vi "RT Train PID.vi"() -> ()   [LabVIEW 2018]
uses:
  <vilib>/Platform/TimedLoop/XDataNode/timing_clust.ctl
  <vilib>/Platform/TimedLoop/XDataNode/nitl_modes.ctl
  <vilib>/Platform/TimedLoop/XDataNode/wakeup.ctl
  <vilib>/Analysis/3filter.llb/Filter Passband Type.ctl
  <vilib>/myRIO/Instrument Drivers/Onboard IO/AI/typedefs/AI Reference.ctl
  <vilib>/myRIO/Common/Instrument Driver Framework/Utilities/typedefs/myRIO Generic Hardware Reference.ctl
  <vilib>/myRIO/Common/Instrument Driver Framework/Utilities/typedefs/Hardware Version Enum.ctl
  <vilib>/myRIO/Common/Instrument Driver Framework/Utilities/typedefs/myRIO v1.0 Reference.ctl
  <vilib>/myRIO/Common/Instrument Driver Framework/Utilities/typedefs/Generic FPGA Reference.ctl
  <vilib>/myRIO/Common/Instrument Driver Framework/myRIO v1.0/AI/typedefs/AI Channels List.ctl
  <vilib>/myRIO/Common/Instrument Driver Framework/myRIO v1.0/AI/typedefs/AI Channels Enum.ctl
  <vilib>/myRIO/Common/Instrument Driver Framework/Utilities/typedefs/Analog Scaling Constants List.ctl
  <vilib>/myRIO/Common/Instrument Driver Framework/Utilities/typedefs/Analog Scaling Constants.ctl
  <vilib>/userdefined/High Color/nirio_resource_hc.ctl
  <vilib>/myRIO/Instrument Drivers/Onboard IO/AO/typedefs/AO Reference.ctl
  <vilib>/myRIO/Common/Instrument Driver Framework/myRIO v1.0/AO/typedefs/AO Channels List.ctl
  <vilib>/myRIO/Common/Instrument Driver Framework/myRIO v1.0/AO/typedefs/AO Channels Enum.ctl
  <vilib>/myRIO/Common/Instrument Driver Framework/Utilities/vis/Is FPGA Ref Available.vi
  <vilib>/myRIO/Common/Instrument Driver Framework/ELVIS III v1.0/AI/vis/ELVIS III v1.1 Open AI.vi
  <vilib>/myRIO/Instrument Drivers/Onboard IO/AI/vis/Read.vi
  6108935b-3925-4b35-9418-db60e5ea9904.vi
  <vilib>/myRIO/Common/Instrument Driver Framework/ELVIS III v1.0/AO/vis/ELVIS III v1.1 Open AO.vi
  <vilib>/myRIO/Instrument Drivers/Onboard IO/AO/vis/Write.vi
  <vilib>/myRIO/Common/Instrument Driver Framework/Utilities/vis/Validate Channels.vi
  <vilib>/myRIO/Common/Instrument Driver Framework/ELVIS III v1.0/AI/vis/ELVIS III v1.0 Reserve AI.vi
  <vilib>/myRIO/Common/Instrument Driver Framework/ELVIS III v1.0/AO/vis/ELVIS III v1.0 Reserve AO.vi
  <vilib>/myRIO/Common/Instrument Driver Framework/ELVIS III v1.0/Resource Manager/vis/ELVIS III v1.0 Reserve Channel List.vi
  <vilib>/myRIO/Common/Instrument Driver Framework/ELVIS III v1.0/AI/vis/ELVIS III v1.0 Build MUX Configuration AI.vi
  <vilib>/myRIO/Common/Instrument Driver Framework/ELVIS III v1.0/AO/vis/ELVIS III v1.0 Build MUX Configuration AO.vi
  <vilib>/myRIO/Common/Instrument Driver Framework/ELVIS III v1.0/Resource Manager/vis/ELVIS III v1.0 Reserve Channel.vi
  <vilib>/myRIO/Common/Instrument Driver Framework/ELVIS III v1.0/Resource Manager/vis/ELVIS III v1.0 Unreserve Channel.vi
  <vilib>/myRIO/Common/Instrument Driver Framework/ELVIS III v1.0/Resource Manager/vis/ELVIS III v1.0 Build Mutex Name.vi
  <vilib>/Utility/VariantDataType/GetNumericInfo.vi
  <vilib>/Utility/error.llb/Error Cluster From Error Code.vi
  <vilib>/myRIO/Common/Instrument Driver Framework/ELVIS III v1.0/ELVIS III v1.1 Open.vi
  <vilib>/myRIO/Common/Instrument Driver Framework/Utilities/vis/IO Manager.vi
  <vilib>/myRIO/Common/Instrument Driver Framework/Utilities/vis/Configuration Manager.vi
  <vilib>/myRIO/Common/Instrument Driver Framework/myRIO v1.0/myRIO v1.0 Close.vi
  <vilib>/myRIO/Common/Instrument Driver Framework/ELVIS III v1.0/AO/vis/ELVIS III v1.0 Write AO.vi
  <vilib>/addons/control/pid/pid.llb/PID (DBL).vi
  <vilib>/myRIO/Common/Instrument Driver Framework/ELVIS III v1.0/Resource Manager/vis/ELVIS III v1.0 Coerce AI Scaling.vi
  <vilib>/myRIO/Common/Instrument Driver Framework/ELVIS III v1.0/Resource Manager/vis/ELVIS III v1.0 Configure AI Mode.vi
  <vilib>/myRIO/Common/Instrument Driver Framework/ELVIS III v1.0/AI/vis/ELVIS III v1.0 Read AI.vi
  <vilib>/myRIO/Express VI/Onboard IO/AO/AO Express VI.xnode
  <vilib>/myRIO/Instrument Drivers/Onboard IO/AO/vis/myRIO AO Open.xnode
  <vilib>/platform/TimedLoop/XDataNode/XDataNode.xnode
  <vilib>/myRIO/Express VI/Onboard IO/AI/AI Express VI.xnode
  <vilib>/myRIO/Instrument Drivers/Onboard IO/AI/vis/myRIO AI Open.xnode
  <vilib>/addons/control/pid/NI_PID_pid.lvlib
  <vilib>/myRIO/Instrument Drivers/Onboard IO/AO/AO.lvlib
  <vilib>/Platform/TimedLoop/XDataNode/XDNodeRunTimeDep.lvlib
  <vilib>/Analysis/NI_AALBase.lvlib
  <vilib>/ptbypt/NI_PtbyPt.lvlib
  <vilib>/myRIO/Instrument Drivers/Onboard IO/AI/AI.lvlib
panel:
  out "B/AI0":dbl(graph)=0.7093639373779297
  out "Finished Late? [i-1] 2":bool
  out "Decoding Freq Detected (B/AI0)":dbl
  out "x/y":dbl=19.0
  out "Detected String":string
  out "Filtered x":dbl(graph)=-0.11171482062742988
  out "Waveform Graph":waveform(dbl)(graph)={"t0"=timestamp(0 s since 1904-01-01), "dt"=2.5, "Y"=[-2.6364378286485904e-06, -5.2778681332887555e-06, -5.293002316547237e-06, -5.317776902443678e-06, -5.350258521277305e-06, -5.397414782842749e-06, -5.47703199116228e-06, -5.552902467398846e-06, -5.7722395439096324e-06, -5.373431116146669e-06, -5.386215220318056e-06, -6.513643938719463e-06, -7.206381354992761e-06, -6.957697945416247e-06, -5.20819315428201e-06, -4.907539706325602e-06, -5.342779616442927e-06, -1.5491993888406056e-05, -1.3042126756574936e-05, -7.539768489912736e-06, 4.004107617116923e-06, -1.4456548126788351e-05, -7.892235984219433e-05, -7.637491547653651e-05, 0.09589586463887334, 2.6726047594847213e-05, -0.00022745795206519749, -0.00030536200943692097, 1.7970273220560155e-05, -0.00033587153778810594, -0.00039858259952325567, -0.0005940095946145293, 0.002812349916099601, -0.0012484148295970718, -0.0011673192539633243, 0.0005959456656431409, -0.0001541859147569749, -0.0007269228170091184, 0.00023360493002714156, -5.086730088528285e-05, 0.003916558554223001, -0.0012346857181189121, 4.4526978413164236e-05, -0.0007204659783994206, 0.00015846422244300714, -0.0004203387420831825, 0.0001334164523498464, -0.0002656047387720224, 0.06336820481823349, -6.069607068970545e-06, 2.9497667763850256e-05, -9.75505327534558e-05, 5.577012061089352e-05, -0.00034639579578911125, -0.0003149596433794245, -0.0002480082718579933, 0.02186898371909846, 9.845455109435623e-05, -0.0004883943445754741, 0.00020141606043958367, 0.00022921410596546307, 0.0006207417465258055, -0.00039600650637702816, -0.00021523328405680445, 0.0015771477242665652, 7.772946215588639e-06, -5.420583580426994e-05, 0.00015345097432138027, -0.0001089926533189178, 0.0007420727345393694, -8.269557920809103e-05, 0.00032844983236722357, 0.10834677049357913, -3.525660349664914e-06, -0.0004681563314324504, 0.00014047742554068962, 0.0003361341823051071, 2.6456586516236954e-05, -0.00044782968840163904, -0.00011287224151005765, 0.002650544784604039, -8.709043451517672e-05, -4.2649930684707325e-05, 0.0002670136466597671, 9.925699441749866e-05, -0.00013402742900023903, 0.00023763672538416232, -0.0002834835661648871, 0.004362910677837028, -3.0818270813087073e-06, -0.0010026600557992448, 0.0010921829218016078, 0.0005029488215995732, 0.00026123852544562544, 6.167950629979222e-05, 0.00019825874036070974, 0.0452660205337438, -0.00035437819761811537, -5.975946168425587e-05, -0.000257283305228602]}
  out "max(x,y)":dbl=0.3379694912310262
  out "Frequencies 2":dbl[](graph)=[195.0]
  # "stop buttons are only for debugging; this will be a startup app"
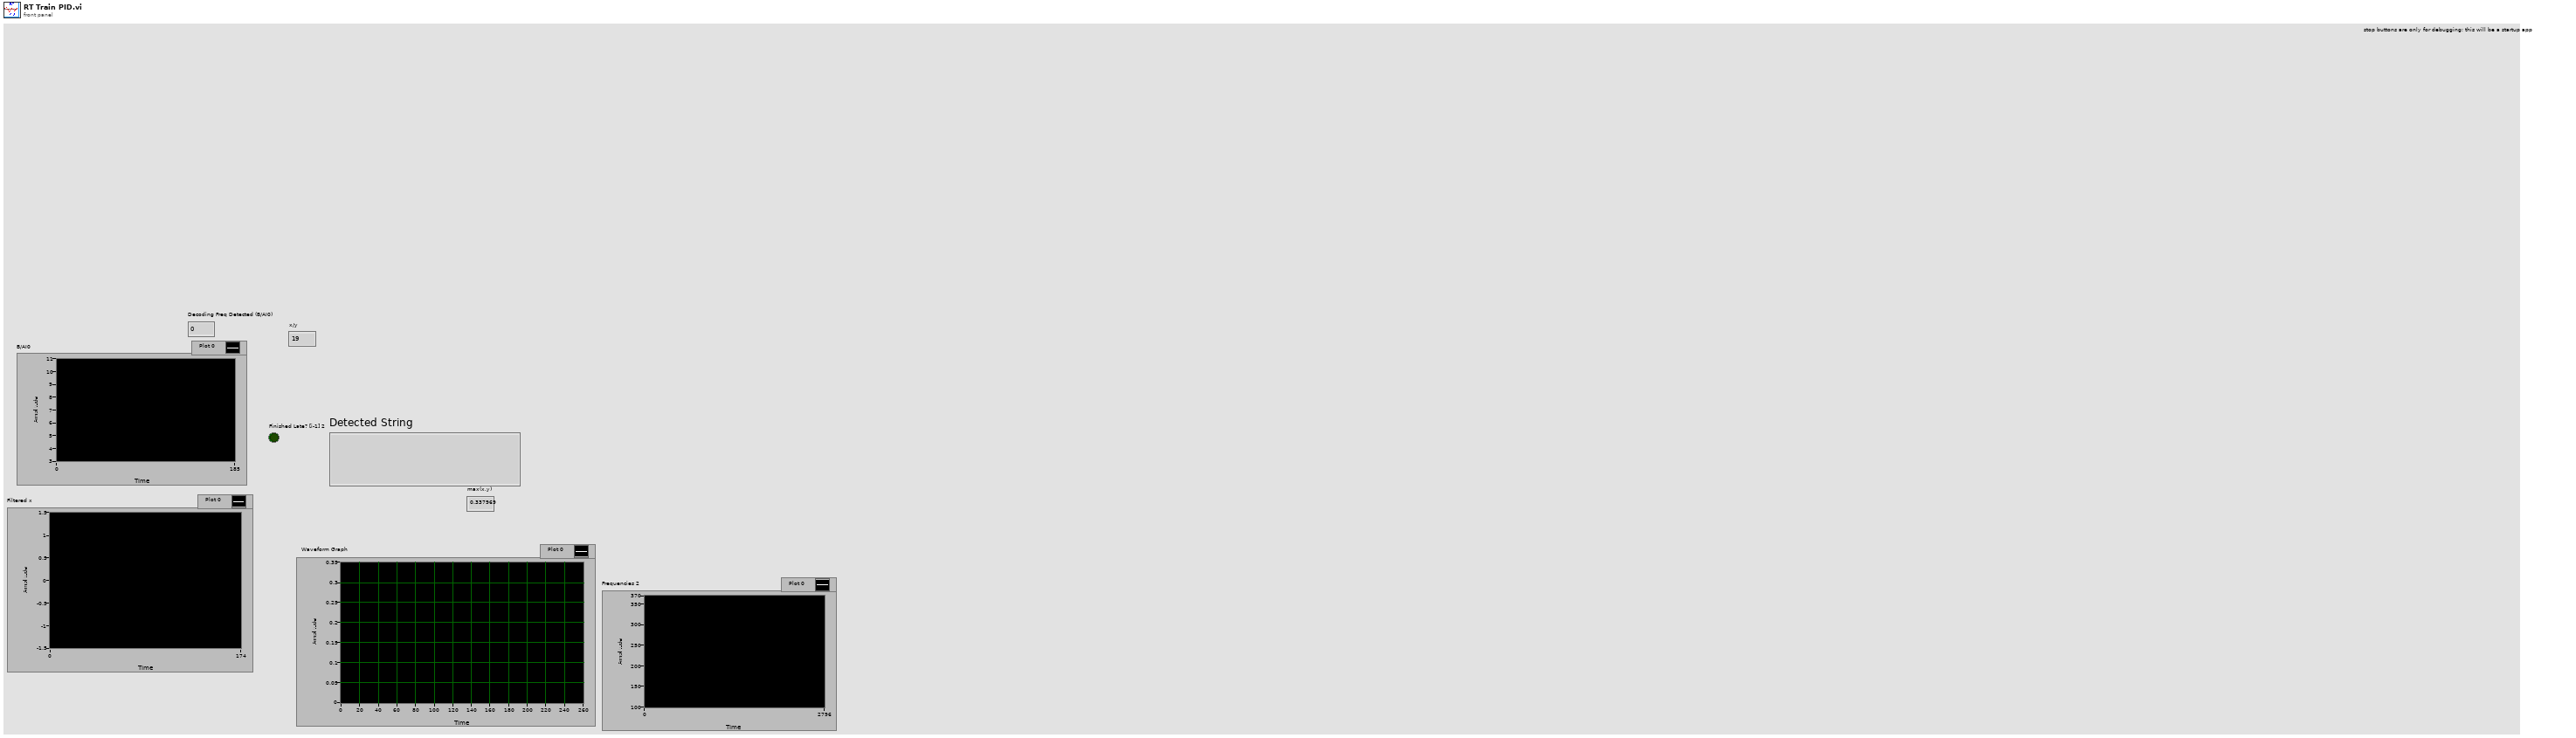
[diagram p1: front panel]
types:
  T1 = typedef "XDNodeRunTimeDep.lvlib/timing_clust.ctl" = cluster{"Expected End [f-1]":u64, "Actual End [f-1]":u64, "Finished Late? [f-1]":bool, "Expected End [i-1]":u64, "Actual End [i-1]":u64, "Finished Late? [i-1]":bool, "Expected Start [i]":u64, "Actual Start [i]":u64, "Expected Start [f]":u64, "Actual Start [f]":u64, "Source Name":string, "Structure Name":string, "Period":i64, "Deadline":i64, "Offset":i64, "Start":i64, "Priority":i32, "Timeout":i32, "Mode":T2, "Wakeup Reason":T3, "Error":errorcluster, "Source Type":string, "Secondary Source Type":string, "Global End Time":u64, "Global Start Time":u64, "Frame Duration":u64, "Iteration Duration":u64, "Assigned CPU":i32, "I/O Scan Engine Mode":u32}
  T2 = typedef "XDNodeRunTimeDep.lvlib/nitl_modes.ctl" = enum32{"No Change", "Process missed periods, maintain original phase", "Discard missed periods, maintain original phase", "Process missed periods, ignore original phase", "Discard missed periods, ignore original phase"}
  T3 = typedef "XDNodeRunTimeDep.lvlib/wakeup.ctl" = enum32{"Normal", "Aborted", "Asynchronous wakeup", "Timing source error", "Timed loop error", "Timeout"}
  T4 = typedef "NI_AALBase.lvlib/Filter Passband Type.ctl" = enum32{"Lowpass", "Highpass", "Bandpass", "Bandstop"}
  T5 = typedef "AI.lvlib/AI Reference.ctl" = cluster{"myRIO Reference":T6, "AI Channels List":T10, "AI Scaling Constants List":T12}
  T6 = typedef "myRIO Generic Hardware Reference.ctl" = cluster{"myRIO Model":T7, "myRIO Hardware Reference":T8}
  T7 = typedef "Hardware Version Enum.ctl" = enum16{"Unknown", "myRIO-1900", "myRIO-1950", "roboRIO", "NI ELVIS RIO CM", "ELVIS III"}
  T8 = typedef "myRIO v1.0 Reference.ctl" = cluster{"Generic FPGA Reference":T9, "Allow multiple opens":bool}
  T9 = typedef "Generic FPGA Reference.ctl" = refnum<k20>
  T10 = typedef "AI Channels List.ctl" = T11[]
  T11 = typedef "AI Channels Enum.ctl" = enum16{"Not Connected", "AudioIn/Left", "AudioIn/Right", "C/AI0", "C/AI1", "A/AI0", "A/AI1", "A/AI2", "A/AI3", "A/AI4", "A/AI5", "A/AI6", "A/AI7", "B/AI0", "B/AI1", "B/AI2", "B/AI3", "B/AI4", "B/AI5", "B/AI6", "B/AI7", "AI/AI0", "AI/AI1", "AI/AI2", "AI/AI3", "A/AI0 (DIFF)", "A/AI1 (DIFF)", "A/AI2 (DIFF)", "A/AI3 (DIFF)", "B/AI0 (DIFF)", "B/AI1 (DIFF)", "B/AI2 (DIFF)", "B/AI3 (DIFF)"}
  T12 = typedef "Analog Scaling Constants List.ctl" = T13[]
  T13 = typedef "Analog Scaling Constants.ctl" = cluster{"LSB Weight (Volts)":dbl, "Offset (Volts)":dbl, "Signed?":bool}
  T14 = typedef "nirio_resource_hc.ctl" = tag
  T15 = typedef "AO.lvlib/AO Reference.ctl" = cluster{"myRIO Reference":T6, "AO Channel List":T16, "AO Scaling Constant List":T12}
  T16 = typedef "AO Channels List.ctl" = T17[]
  T17 = typedef "AO Channels Enum.ctl" = enum16{"Not Connected", "AudioOut/Left", "AudioOut/Right", "C/AO0", "C/AO1", "A/AO0", "A/AO1", "B/AO0", "B/AO1"}
  T18 = cluster{"proportional gain (Kc)":dbl, "integral time (Ti, min)":dbl, "derivative time (Td, min)":dbl}
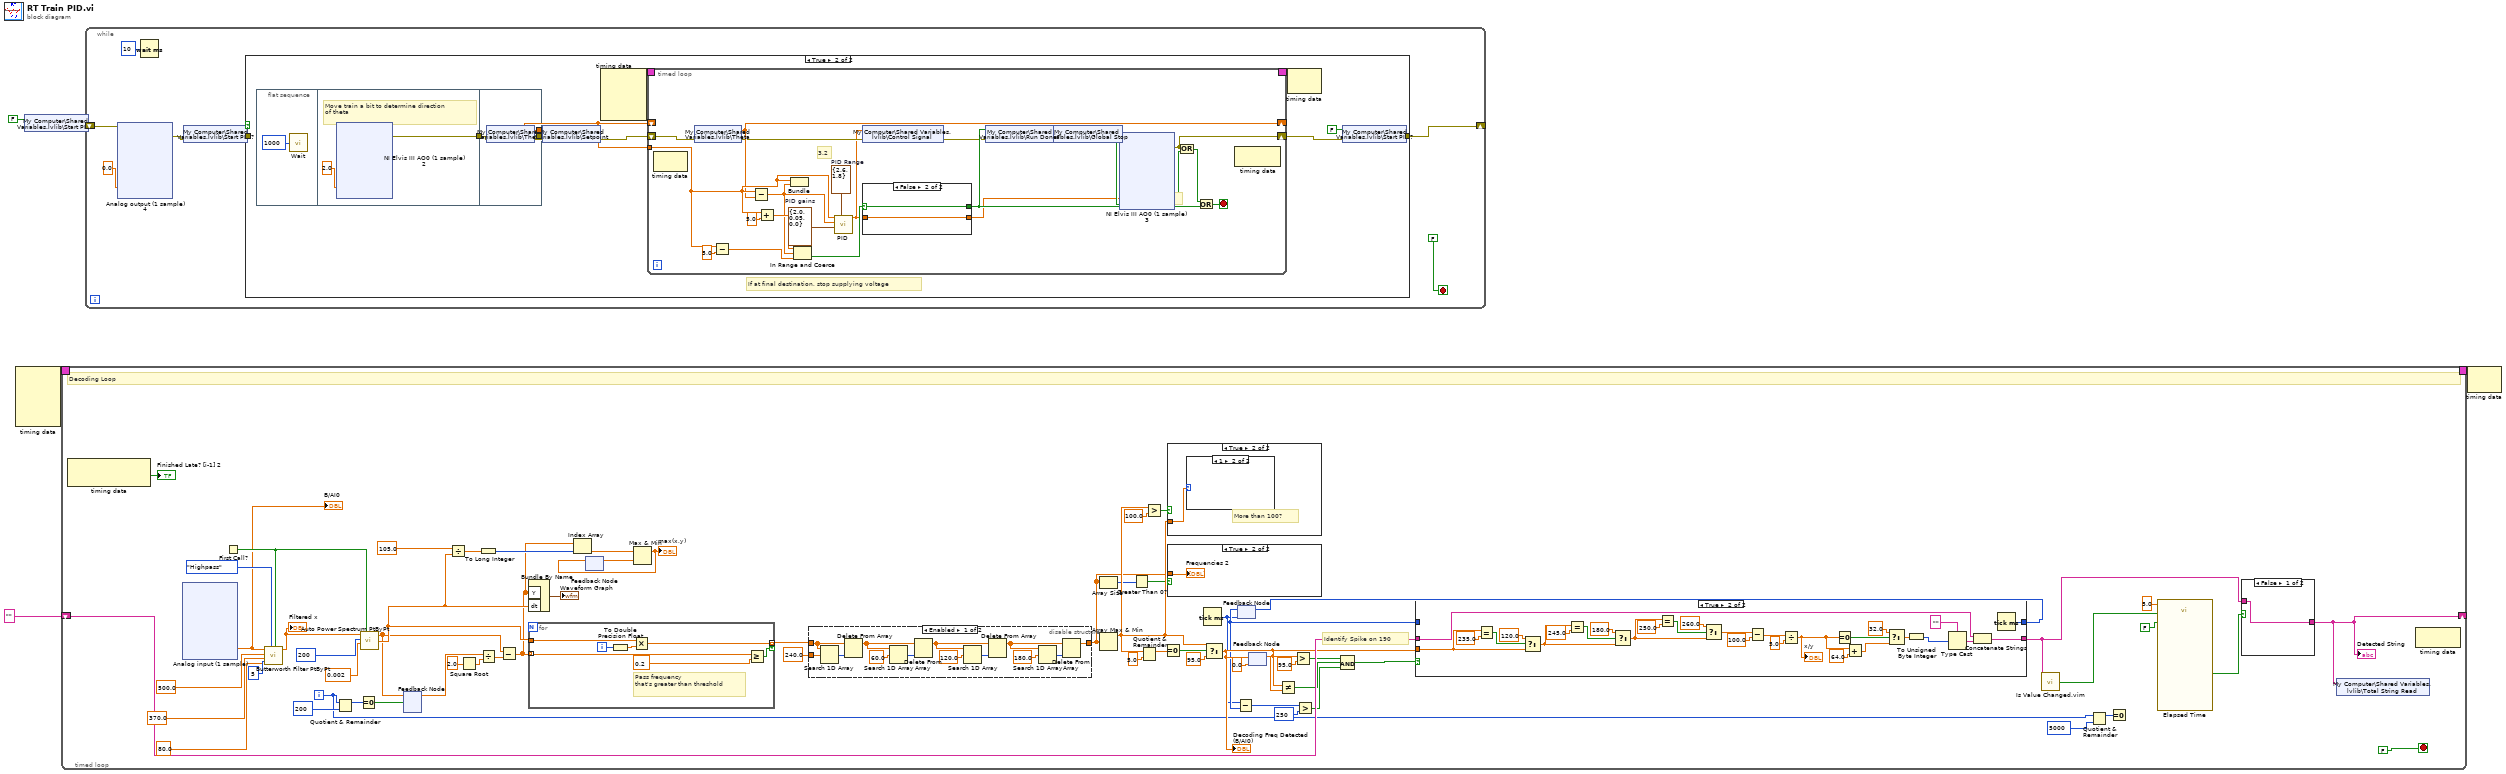
[diagram p0: block diagram]
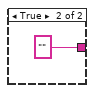
[diagram p2: hidden frame]
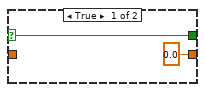
[diagram p9: hidden frame]
diagram:
  n1 = node-c288() -> (w3:T1)  [unwired: 5 in]
  n2 = shared-variable "My Computer\\Shared Variables.lvlib\\Start PID?"(FALSE ("Start PID?")) -> (error out=w4:errorcluster)  [unwired: 1 in]
  n3 = timed-loop {
    timing: w3 -> [_]
    timing-out: [_] -> w2
    shift-right: [w6] -> _
    shift-left: "" -> [w51]
    i -> [w14]
    stop <- FALSE stop-if-true
    # "Identify Spike on 190"
    # "Decoding Loop"
    n4 = node-c288() -> (→"Finished Late? [i-1] 2":bool)  [unwired: 1 in, 1 out]
    n5 = xnode "Analog input (1 sample)"() -> ("B/AI0 (DIFF)"=w15:dbl)  [unwired: 1 in, 1 out]
    "B/AI0" <- w15
    n6 = First Call?() -> (First Call?: T/F=w50:bool)
    n7 = call <vilib>:"Butterworth Filter PtByPt.vi"("initialize"=w50, "order"=5, "filter type"=Filter_Passband_Type."Highpass", "low cutoff freq: fl"=80.0, "high cutoff freq: fh"=370.0, "sampling freq: fs"=500.0, "x"=w15) -> ("Filtered x"=w49:dbl)  [unwired: 2 in, 1 out]
    "Filtered x" <- w49
    n8 = Quotient & Remainder(x=w14, y=200) -> (x-y*floor(x/y)=w26:i32)  [unwired: 1 out]
    n9 = Equal To 0?(x=w26) -> (x = 0?=w25:bool)
    n10 = call <vilib>:"Auto Power Spectrum PtByPt.vi"("signal"=w49, "sample length"=200 ("sample length 2"), "dt"=0.002, "initialize"=w50) -> ("Power Spectrum (V^2 rms)"=w21:dbl[], "df"=w62:dbl)  [unwired: 1 in, 1 out]
    n11 = feedback-in #1(w21, w25) -> ()
    n12 = feedback #1() -> (w30:dbl[])  [unwired: 1 in]
    n13 = Divide(x=105.0 ("Freq to Set 2"), y=w62) -> (x/y=w64:dbl)
    n14 = Square Root(x=2.0) -> (sqrt(x)=w28:dbl)
    n15 = To Long Integer(number=w64) -> (32bit integer=w63:i32)
    n16 = Divide(x=w30, y=w28) -> (x/y=w27:dbl[])
    n17 = Subtract(x=w21, y=w27) -> (x-y=w20:dbl[])
    n18 = Bundle By Name("Y"=w20, "dt"=w62) -> (→"Waveform Graph":waveform(dbl))  [unwired: 1 in]
    n19 = for {
      tunnel: [w118] -> w39 mode=indexing if=w123
      tunnel: w20 -> [w119] mode=indexing
      tunnel: w62 -> [w122]
      i -> [w121]
      # "Pass frequency\nthat's greater than threshold"
      n20 = To Double Precision Float(number=w121) -> (double precision float=w120:dbl)
      n21 = Multiply(x=w122, y=w120) -> (x*y=w118:dbl)
      n22 = Greater Or Equal?(x=w119, y=0.2) -> (x >= y?=w123:bool)
    }
    n23 = Index Array(array=w20, index=w63) -> (element=w36:dbl)
    n24 = feedback #2() -> (w38:dbl)  [unwired: 1 in]
    n25 = Max & Min(x=w36, y=w38) -> (max(x,y)=w37:dbl)  [unwired: 1 out]
    "max(x,y)" <- w37
    n26 = feedback-in #2(w37) -> ()
    n27 = disable-structure shown="Enabled" {
      disable-tunnel: 240.0 ("element") -> [w85 _]
      disable-tunnel: w39 -> [w84 w86]
      disable-tunnel: [w73 w86] -> w17
      frame Enabled {
        n28 = Search 1D Array(1D array=w84, element=w85) -> (index of element=w80:i32)  [unwired: 1 in]
        n29 = Delete From Array(array=w84, index=w80) -> (array with subset deleted=w81:dbl[])  [unwired: 1 in, 1 out]
        n30 = Search 1D Array(1D array=w81, element=60.0) -> (index of element=w83:i32)  [unwired: 1 in]
        n31 = Delete From Array(array=w81, index=w83) -> (array with subset deleted=w77:dbl[])  [unwired: 1 in, 1 out]
        n32 = Search 1D Array(1D array=w77, element=120.0) -> (index of element=w78:i32)  [unwired: 1 in]
        n33 = Delete From Array(array=w77, index=w78) -> (array with subset deleted=w74:dbl[])  [unwired: 1 in, 1 out]
        n34 = Search 1D Array(1D array=w74, element=180.0) -> (index of element=w76:i32)  [unwired: 1 in]
        n35 = Delete From Array(array=w74, index=w76) -> (array with subset deleted=w73:dbl[])  [unwired: 1 in, 1 out]
      }
      frame Disabled {
      }
    }
    n36 = Array Size(array=w17) -> (size(s)=w18:i32)
    n37 = Array Max & Min(array=w17) -> (max value=w23:dbl)  [unwired: 3 out]
    n38 = Greater Than 0?(x=w18) -> (x > 0?=w19:bool)
    n39 = Quotient & Remainder(x=w23, y=5.0) -> (x-y*floor(x/y)=w55:dbl)  [unwired: 1 out]
    n40 = Greater?(x=w23, y=100.0) -> (0:w60:bool)
    n41 = Equal To 0?(x=w55) -> (x = 0?=w54:bool)
    n42 = case shown="True" w60 {
      tunnel: w23 -> [_ w117]
      frame False {
      }
      frame True {
        # "More than 100?"
        n43 = case shown="1" w117 {
          frame 0, Default {
          }
          frame 1 {
          }
        }
      }
    }
    n44 = case shown="True" w19 {
      tunnel: w17 -> [_ w72]
      frame False {
      }
      frame True {
        "Frequencies 2" <- w72
      }
    }
    n45 = Tick Count (ms)() -> (millisecond timer value=w31:u32)
    n46 = Select(t=w23, s=w54, f=95.0) -> (s? t:f=w44:dbl)
    "Decoding Freq Detected (B/AI0)" <- w44
    n47 = feedback #3(w31) -> (w34:u32)
    n48 = Subtract(x=w31, y=w34) -> (x-y=w33:u32)
    n49 = feedback-in #4(w44) -> ()
    n50 = feedback #4(0.0 ("f")) -> (w42:dbl)
    n51 = Not Equal?(x=w44, y=w42) -> (x != y?=w46:bool)
    n52 = Greater?(x=w44, y=95.0) -> (0:w47:bool)
    n53 = Greater?(x=w33, y=u32 250) -> (0:w22:bool)
    n54 = Compound Arithmetic op=AND(w47, w46, w22) -> (w45:bool)
    n55 = case shown="True" w45 {
      tunnel: w44 -> [_ w103]
      tunnel: [w88 w108] -> w7
      tunnel: w51 -> [w88 w110]
      tunnel: [w87 w107] -> w35
      tunnel: w34 -> [w87 _]
      frame False {
      }
      frame True {
        n56 = Equal?(x=w103, y=235.0) -> (x = y?=w106:bool)
        n57 = Select(t=120.0, s=w106, f=w103) -> (s? t:f=w99:dbl)
        n58 = Equal?(x=w99, y=245.0) -> (x = y?=w101:bool)
        n59 = Select(t=180.0, s=w101, f=w99) -> (s? t:f=w95:dbl)
        n60 = Equal?(x=w95, y=250.0) -> (x = y?=w97:bool)
        n61 = Select(t=260.0, s=w97, f=w95) -> (s? t:f=w89:dbl)
        n62 = Subtract(x=w89, y=100.0) -> (x-y=w115:dbl)
        n63 = Divide(x=w115, y=5.0) -> (x/y=w90:dbl)
        "x/y" <- w90
        n64 = Equal To 0?(x=w90) -> (x = 0?=w94:bool)
        n65 = Add(x=w90, y=64.0) -> (x+y=w92:dbl)
        n66 = Select(t=32.0, s=w94, f=w92) -> (s? t:f=w91:dbl)
        n67 = To Unsigned Byte Integer(number=w91) -> (unsigned 8bit integer=w111:u8)
        n68 = Type Cast(type="", x=w111) -> (*(type *) &x=w109:string)
        n69 = Concatenate Strings(w110, w109) -> (w108:string)
        n70 = Tick Count (ms)() -> (millisecond timer value=w107:u32)
      }
    }
    n71 = feedback-in #3(w35) -> ()
    n72 = call "Is Value Changed.vim"("value"=w7) -> ("changed or first call?"=w10:bool)
    n73 = Quotient & Remainder(x=w14, y=5000) -> (x-y*floor(x/y)=w12:i32)  [unwired: 1 out]
    n74 = Equal To 0?(x=w12) -> ()  [unwired: 1 out]
    n75 = call "Elapsed Time"("Time Target (s)"=5.0, "Reset"=w10, "Auto Reset"=FALSE) -> ("Time has Elapsed"=w8:bool)  [unwired: 9 in, 7 out]
    n76 = case shown="False" w8 {
      tunnel: [w70 ""] -> w6
      tunnel: w7 -> [w70 _]
      frame False {
      }
      frame True {
      }
    }
    "Detected String" <- w6
    n77 = shared-variable "My Computer\\Shared Variables.lvlib\\Total String Read"(w6) -> ()  [unwired: 1 in, 1 out]
    n78 = node-c288() -> ()  [unwired: 1 in, 1 out]
  }
  n79 = while {
    shift-right: [w175] -> _
    shift-left: w4 -> [w173]
    stop <- FALSE stop-if-true
    n80 = xnode "Analog output (1 sample) 4"("A/AO0"=0.0 ("C/AO0 (AO0)"), "error in (no error)"=w173) -> ("error out"=w174:errorcluster)
    n81 = Wait (ms)(milliseconds to wait=u32 10) -> ()  [unwired: 1 out]
    n82 = shared-variable "My Computer\\Shared Variables.lvlib\\Start PID?"(error in=w174) -> (w177:bool, error out=w176:errorcluster)
    n83 = case shown="True" w177 {
      tunnel: w176 -> [w216 _]
      tunnel: [w216 w217] -> w175
      frame False {
      }
      frame True {
        # "If at final destination, stop supplying voltage"
        n84 = flat-sequence {
          tunnel: [w228] -> w223
          tunnel: [w268] -> w219
          tunnel: [w267] -> w222
          tunnel: w223 -> [w266]
          frame #0 {
            n85 = call "Wait"("Count(mSec)"=u32 1000) -> ()  [unwired: 1 out]
          }
          frame #1 {
            # "Move train a bit to determine direction\nof theta"
            n86 = xnode "NI Elvis III AO0 (1 sample) 2"("A/AO0"=2.0 ("C/AO0 (AO0)")) -> ("error out"=w228:errorcluster)  [unwired: 1 in]
          }
          frame #2 {
            n87 = shared-variable "My Computer\\Shared Variables.lvlib\\Theta"(error in=w266) -> (w268:dbl, error out=w267:errorcluster)
          }
        }
        n88 = shared-variable "My Computer\\Shared Variables.lvlib\\Setpoint"(w219, error in=w222) -> (error out=w218:errorcluster)
        n89 = node-c288() -> (w225:T1)  [unwired: 4 in]
        n90 = timed-loop {
          timing: w225 -> [_]
          timing-out: [_] -> w224
          tunnel: w219 -> [w288]
          shift-right: [w276] -> _
          shift-left: w219 -> [_]
          shift-right: [w271] -> w221
          shift-left: w218 -> [w275]
          stop <- w281 stop-if-true
          w289 = T18 {"proportional gain (Kc)"=2.0, "integral time (Ti, min)"=0.05, "derivative time (Td, min)"=0.0}  # PID gains
          w290 = cluster{"output high":dbl, "output low":dbl} {"output high"=2.6, "output low"=1.8}  # PID Range
          # "3.2"
          # "Make motor go"
          n91 = node-c288() -> ()  [unwired: 1 in, 1 out]
          n92 = shared-variable "My Computer\\Shared Variables.lvlib\\Theta"(error in=w275) -> (w276:dbl, error out=w274:errorcluster)
          n93 = Subtract(x=w288, y=5.0) -> (x-y=w284:dbl)
          n94 = Subtract(x=w288, y=w276) -> (x-y=w277:dbl)
          n95 = Add(x=w288, y=5.0) -> (x+y=w285:dbl)
          n96 = Bundle("Double"=w288, w277) -> ()  [unwired: 1 in, 1 out]
          n97 = In Range and Coerce(upper limit=w285, x=w277, lower limit=w284) -> (In Range?=w283:bool)  [unwired: 1 out]
          n98 = call-poly <vilib>:"PID.vi"("output range"=w290, "PID gains"=w289, "process variable"=w277, "setpoint"=w288) -> ("output"=w273:dbl)  [unwired: 6 in, 1 out]
          n99 = shared-variable "My Computer\\Shared Variables.lvlib\\Control Signal"(w273, error in=w274) -> (error out=w270:errorcluster)
          n100 = case shown="False" w283 {
            selector: w283 -> [w328 w330]
            tunnel: [0.0 ("output") w331] -> w272
            tunnel: w273 -> [_ w331]
            tunnel: [w328 w330] -> w279
            frame True {
            }
            frame False {
            }
          }
          n101 = shared-variable "My Computer\\Shared Variables.lvlib\\Run Done?"(w279, error in=w270) -> (error out=w278:errorcluster)
          n102 = shared-variable "My Computer\\Shared Variables.lvlib\\Global Stop"(error in=w278) -> (w282:bool, error out=w269:errorcluster)
          n103 = xnode "NI Elvis III AO0 (1 sample) 3"("A/AO0"=w272, "error in (no error)"=w269) -> ("error out"=w271:errorcluster)
          n104 = Or(x=w271, y=w282) -> (x .or. y?=w280:bool)
          n105 = Or(x=w280, y=w279) -> (x .or. y?=w281:bool)
          n106 = node-c288() -> ()  [unwired: 1 in, 1 out]
        }
        n107 = node-c288(w224) -> ()  [unwired: 1 out]
        n108 = shared-variable "My Computer\\Shared Variables.lvlib\\Start PID?"(FALSE ("Start PID?"), error in=w221) -> (error out=w217:errorcluster)
      }
    }
  }
  n109 = node-c288(w2) -> ()  [unwired: 1 out]
